vi "HydAcqMaster.vi"() -> ()   [LabVIEW 2022 SP3]
uses:
  ScanningControl/Digitizers/GaGe/-GageUtils/GageGlobals.vi
  <instrlib>/LeCroy Wave Series/LeCroy Wave Series.lvlib
  <vilib>/Utility/file.llb/Read From Spreadsheet File (DBL).vi
panel:
  in  "Erase Data":bool
  out "size(s)":i32[](array[numeric])
  out "Hydrophone Calibration Data":sgl[][](array[numeric]) format="%0.3f"
  out "Calibration Data in use":sgl[](array[numeric])
  in  "Frequency of Interest":u16(ring) items=["1", "2", "3", "4", "5", "6", "7", "8", "9", "10", "11", "12", "13", "14", "15"]
  in  "Hydrophone File":u16(ring) items=["Hydrophone001.txt", "Hydrophone006.txt", "Hydrophone007.txt", "Hydrophone009.txt", "Hydrophone010.txt", "Hydrophone011.txt", "Hydrophone012.txt", "Hydrophone013.txt", "Hydrophone014.txt", "Hydrophone015.txt", "Hydrophone016.txt", "Hydrophone017.txt", "Hydrophone018.txt"]
  in  "LeCroy IP":refnum<visa-resource-name>="VICP::172.25.2.101"
  in  "View Data":bool
  in  "Comment field":string
  in  "Save path":path=path "C:/"
  in  "Scope":bool
  in  "Amp (kV)":sgl
  in  "Init?":bool=TRUE
  out "Handle Cluster 2":T1
  out "Handle Cluster":T1
  in  "FileName":string="test"
  in  "Save Data":bool
  out "Waveforms":sgl[][](graph)
  in  "Sequence":u16=1
  out "Peak Values":cluster{"Z Element Position":sgl[], sgl[]}[](graph)
  in  "Time Out (ms)":dbl=1000.0 min=-1.0
  in  "# Firings":u16=1 min=1
  in  "start scan":bool
  in  "SetDig":bool
  in  "ExitSendCmd":bool
  # "© 2012 Riverside Research Institute"
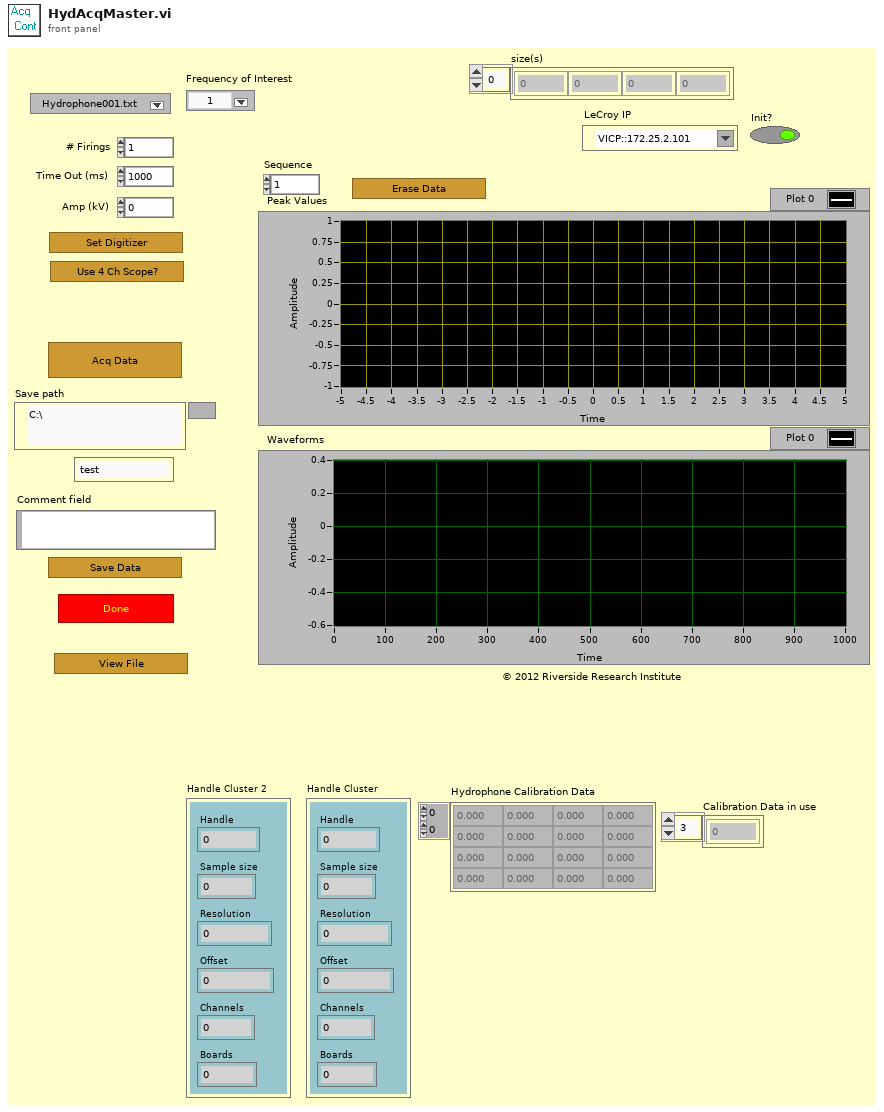
[diagram p1: front panel]
types:
  T1 = cluster{"Handle":u32, "Sample size":u32, "Resolution":i32, "Offset":i32, "Channels":u32, "Boards":u32}
  T2 = enum16{"open", "replace", "create", "open or create", "replace or create", "replace or create with confirmation"}
  T3 = enum16{"big-endian, network order", "native, host order", "little-endian"}
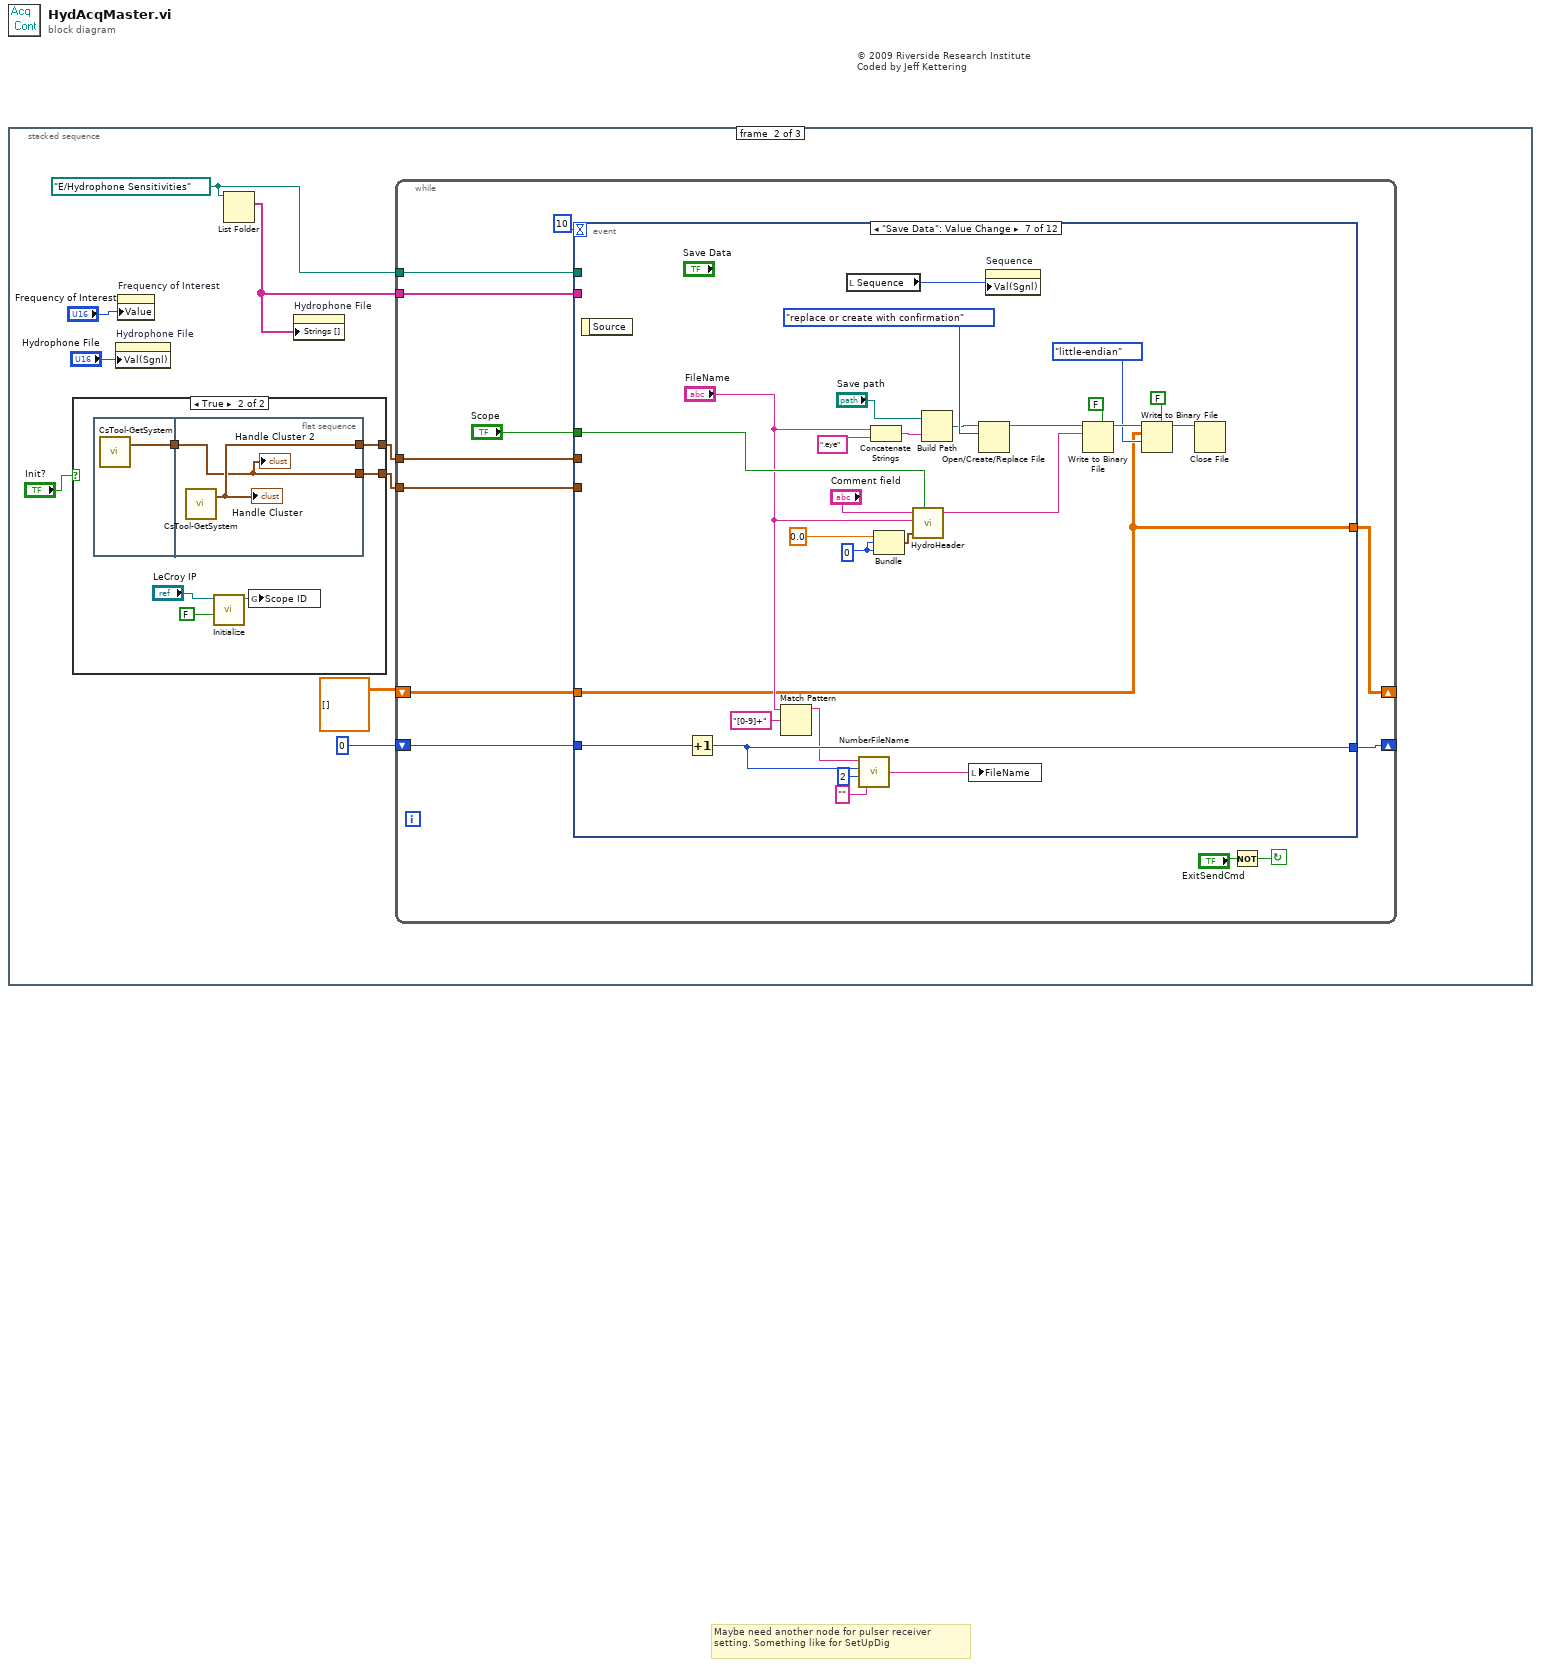
[diagram p0: block diagram]
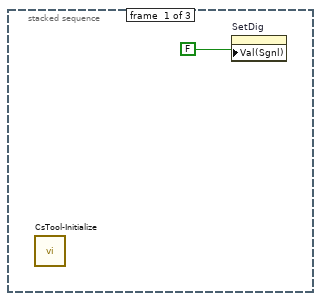
[diagram p2: hidden frame]
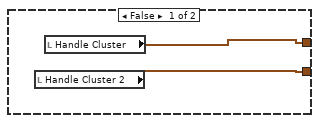
[diagram p3: hidden frame]
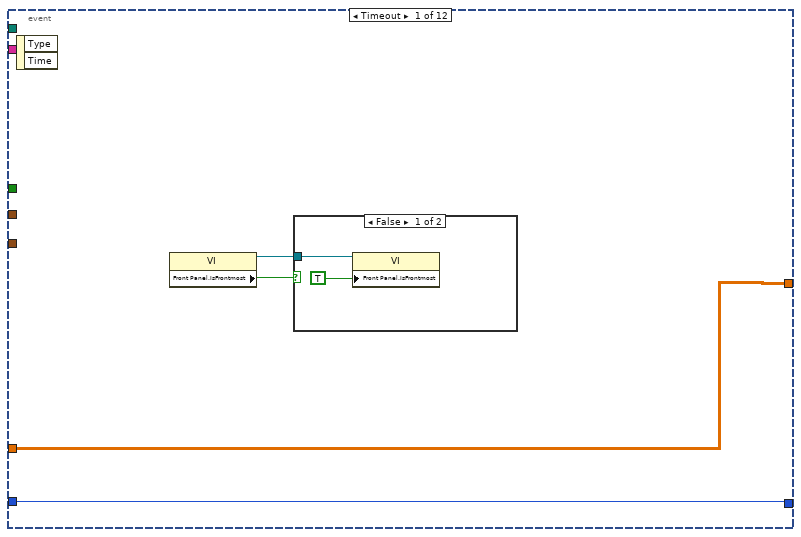
[diagram p4: hidden frame]
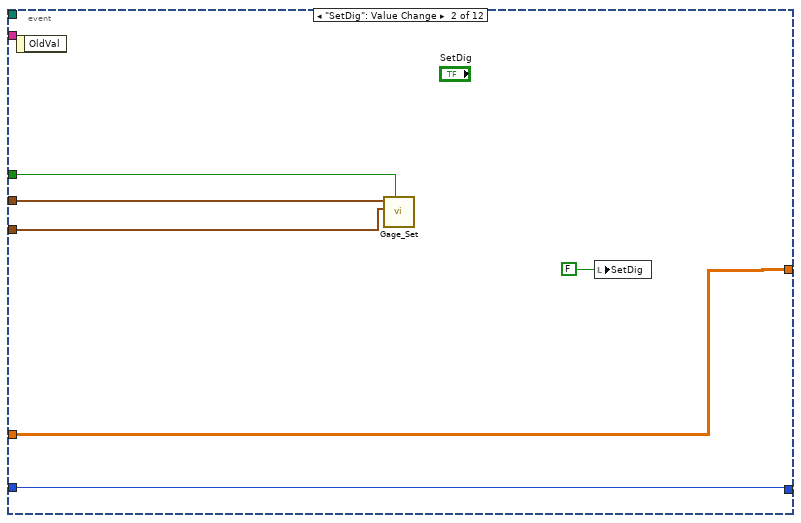
[diagram p6: hidden frame]
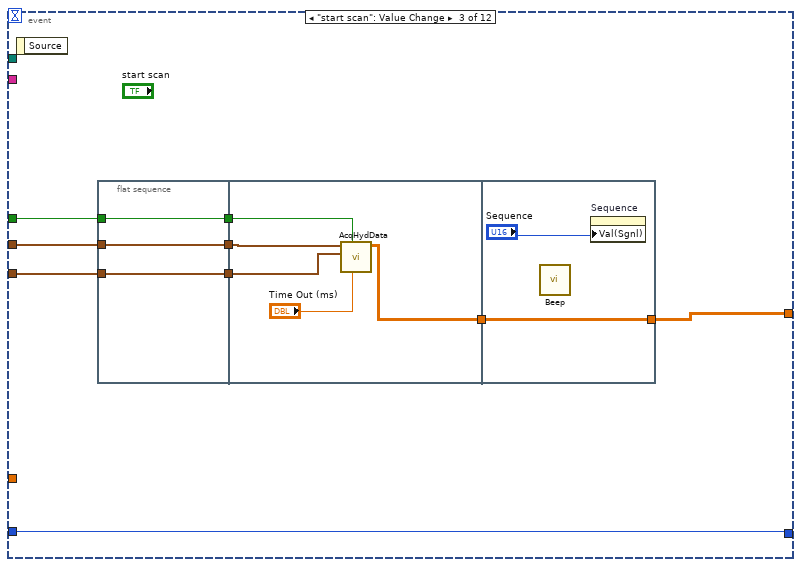
[diagram p7: hidden frame]
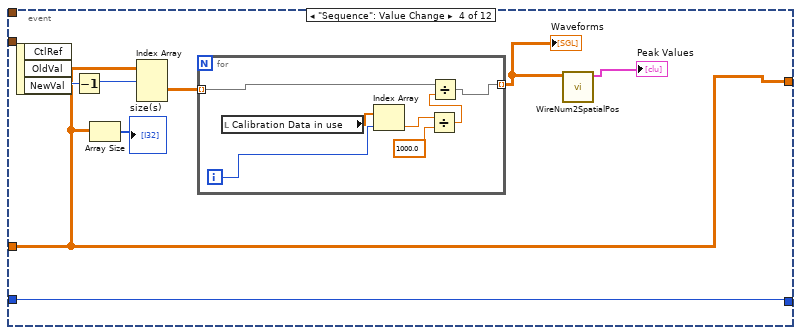
[diagram p8: hidden frame]
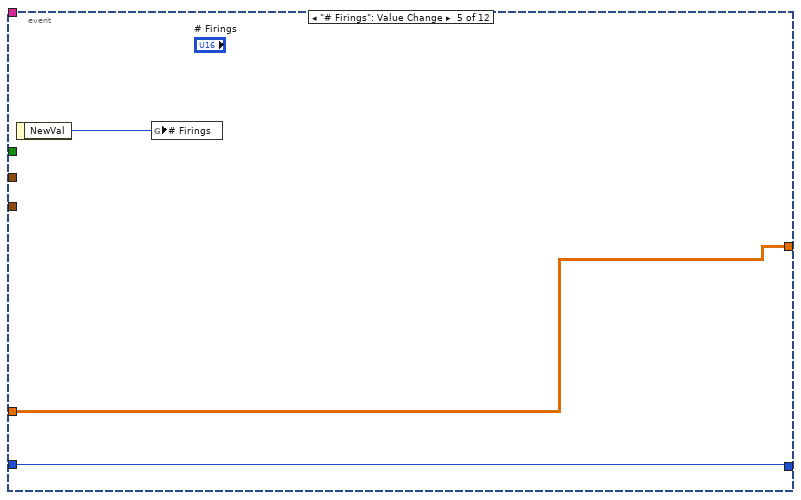
[diagram p9: hidden frame]
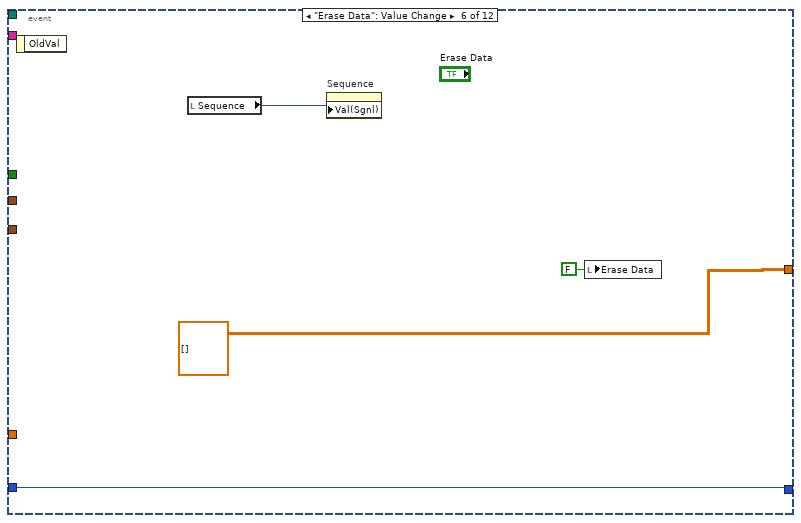
[diagram p10: hidden frame]
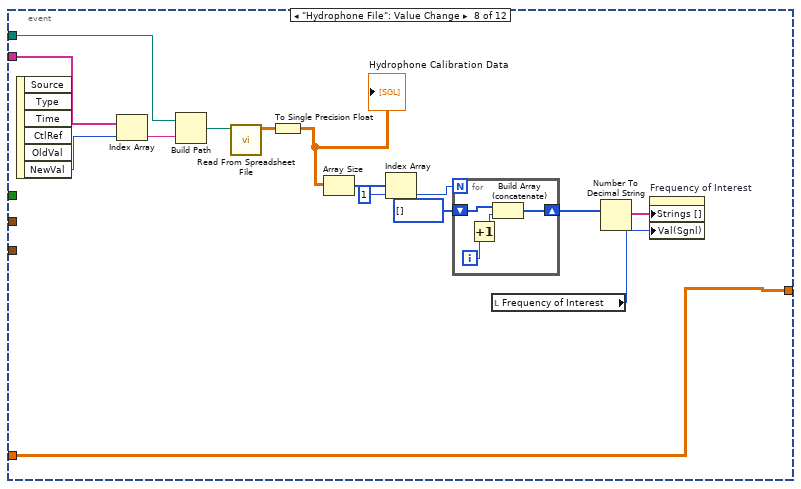
[diagram p11: hidden frame]
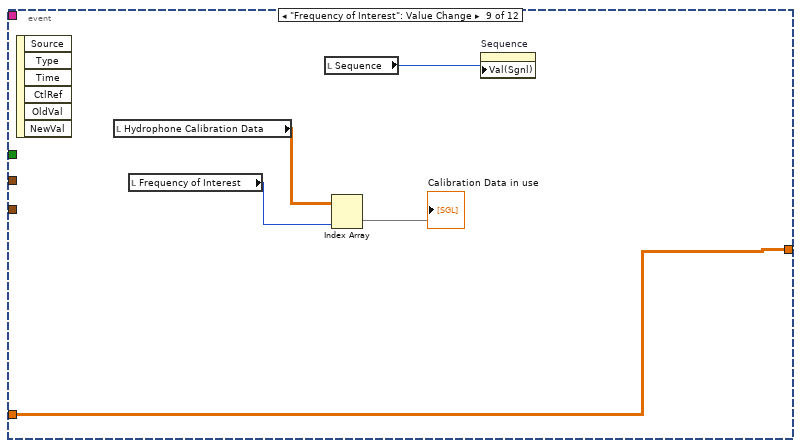
[diagram p12: hidden frame]
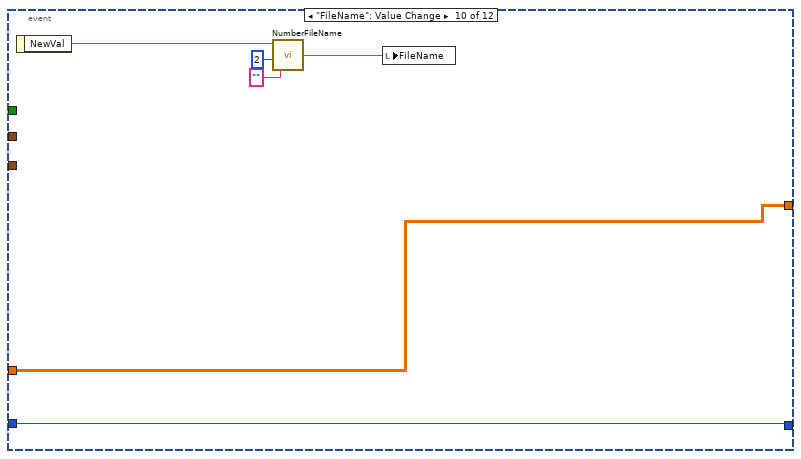
[diagram p13: hidden frame]
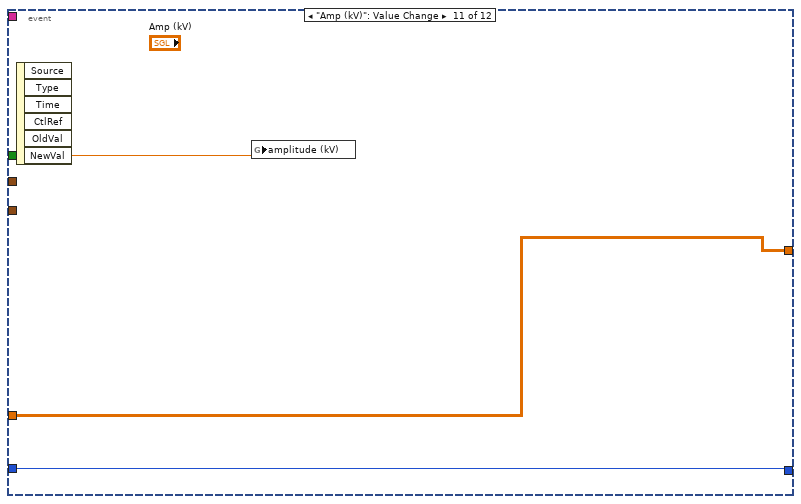
[diagram p14: hidden frame]
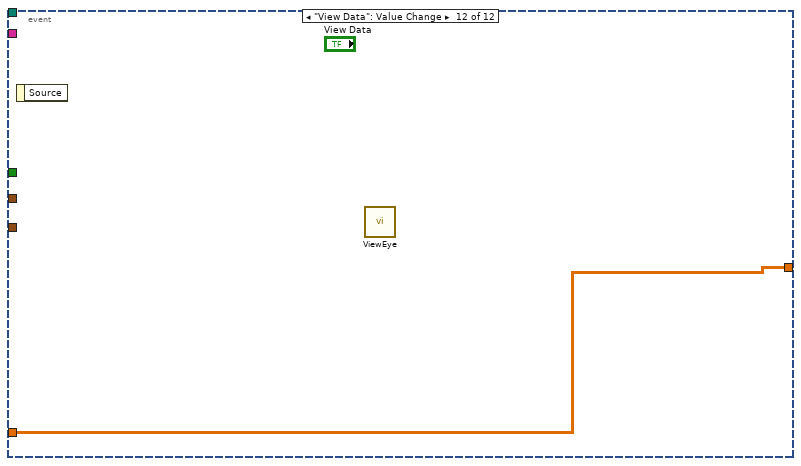
[diagram p15: hidden frame]
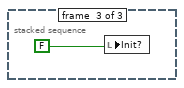
[diagram p16: hidden frame]
diagram:
  # "© 2009 Riverside Research Institute\nCoded by Jeff Kettering"
  # "Maybe need another node for pulser receiver setting. Something like for SetUpDig"
  n1 = stacked-sequence {
    frame #0 {
      n2 = call <userlib>:"CsTool-Initialize.vi"() -> ()  [unwired: 2 out]
      n3 = property on="SetDig" class="Bool (strict)"("Val(Sgnl)"=FALSE) -> ()  [unwired: 2 in, 2 out]
    }
    frame #1 {
      w5 = path "E:/Hydrophone Sensitivities" ("path")
      n4 = case shown="True" "Init?" {
        tunnel: [w12 w17] -> w10
        tunnel: [w11 w16] -> w9
        frame False {
          n5 = local read "Handle Cluster 2"() -> (w11:T1)
          n6 = local read "Handle Cluster"() -> (w12:T1)
        }
        frame True {
          n7 = flat-sequence {
            tunnel: [w19] -> w18
            tunnel: [w21] -> w17
            tunnel: w18 -> [w20]
            tunnel: [w20] -> w16
            frame #0 {
              n8 = call <userlib>:"CsTool-GetSystem.vi"() -> ("Handle Cluster"=w19:T1)  [unwired: 4 in, 1 out]
            }
            frame #1 {
              n9 = call <userlib>:"CsTool-GetSystem.vi"() -> ("Handle Cluster"=w21:T1)  [unwired: 4 in, 1 out]
              "Handle Cluster" <- w21
              "Handle Cluster 2" <- w20
            }
          }
          n10 = call <instrlib>:"Initialize.vi"("Reset? (T: Yes)"=FALSE, "VISA resource name"="LeCroy IP") -> ("VISA resource name out"=w15:refnum<visa-resource-name>)  [unwired: 2 in, 7 out]
          n11 = global write "GageGlobals.vi" "Scope ID"(w15) -> ()
        }
      }
      n12 = property on="Hydrophone File" class="Ring (strict)"("Val(Sgnl)"="Hydrophone File") -> ()  [unwired: 2 in, 2 out]
      n13 = property on="Frequency of Interest" class="Ring (strict)"("Value"="Frequency of Interest") -> ()  [unwired: 2 in, 2 out]
      n14 = List Folder(path=w5) -> (filenames=w2:string[])  [unwired: 3 in, 3 out]
      n15 = property on="Hydrophone File" class="Ring (strict)"("Strings []"=w2) -> ()  [unwired: 2 in, 2 out]
      n16 = while {
        tunnel: w10 -> [w30]
        tunnel: w9 -> [w29]
        shift-right: [w26] -> _
        shift-left: 0 -> [w27]
        tunnel: w2 -> [w25]
        tunnel: w5 -> [w24]
        shift-right: [w23] -> _
        shift-left: sgl[][][] [] ("Data in Volts") -> [w22]
        stop <- w32 continue-if-true
        n17 = event shown="[6] \"Save Data\": Value Change" {
          selector: _ -> [_ _ _ _ _ _ _ _ _ _ _ _]
          dyn-events: _ -> [_ _ _ _ _ _ _ _ _ _ _ _]
          timeout: 10 -> [_ _ _ _ _ _ _ _ _ _ _ _]
          tunnel: w30 -> [_ w45 w54 _ _ _ _ _ _ _ _ _]
          tunnel: w29 -> [_ w44 w53 _ _ _ _ _ _ _ _ _]
          tunnel: "Scope" -> [_ w43 w52 _ _ _ w99 _ _ _ _ _]
          tunnel: w27 -> [w35 w42 w51 w71 w81 w86 w97 _ _ w140 w145 _]
          tunnel: [w35 w42 w51 w71 w81 w86 w94 _ _ w140 w145 _] -> w26
          tunnel: w25 -> [_ _ _ _ _ _ _ w126 _ _ _ _]
          tunnel: w24 -> [_ _ _ _ _ _ _ w124 _ _ _ _]
          tunnel: [w34 w40 w47 w66 w80 sgl[][][] [] ("Data in Volts") w87 w115 w134 w138 w144 w147] -> w23
          tunnel: w22 -> [w34 w40 _ w66 w80 _ w87 w115 w134 w138 w144 w147]
          event Timeout {
            n18 = event-data() -> ()  [unwired: 3 out]
            n19 = property class="VI"() -> (reference out=w37:refnum<vi>, "Front Panel.IsFrontmost"=w36:bool)  [unwired: 2 in, 1 out]
            n20 = case shown="False" w36 {
              tunnel: w37 -> [w39 _]
              frame False {
                n21 = property class="VI"(reference=w39, "Front Panel.IsFrontmost"=TRUE) -> ()  [unwired: 1 in, 2 out]
              }
              frame True {
              }
            }
          }
          event "SetDig": Value Change {
            n22 = event-data() -> ()  [unwired: 2 out]
            n23 = call "Gage_Set.vi"("Scope"=w43, "Handle Cluster 2"=w44, "Handle Cluster 1"=w45) -> ()  [unwired: 9 out]
            n24 = local write "SetDig"(FALSE) -> ()
          }
          event "start scan": Value Change {
            n25 = event-data() -> ()  [unwired: 2 out]
            n26 = flat-sequence {
              tunnel: w52 -> [w55]
              tunnel: w53 -> [w56]
              tunnel: w54 -> [w57]
              tunnel: [w57] -> w50
              tunnel: [w56] -> w49
              tunnel: [w55] -> w48
              tunnel: w50 -> [w62]
              tunnel: w49 -> [w61]
              tunnel: w48 -> [w59]
              tunnel: [w58] -> w46
              tunnel: [w63] -> w47
              tunnel: w46 -> [w63]
              frame #0 {
              }
              frame #1 {
                n27 = call "AcqHydData.vi"("Time Out (ms)"="Time Out (ms)", "Scope"=w59, "Handle Cluster 2"=w61, "Handle Cluster 1"=w62) -> ("Data in Volts"=w58:sgl[][][])  [unwired: 7 out]
              }
              frame #2 {
                n28 = call <vilib>:"Beep.vi"() -> ()  [unwired: 3 in, 9 out]
                n29 = property on="Sequence" class="DigNum (strict)"("Val(Sgnl)"="Sequence") -> ()  [unwired: 2 in, 2 out]
              }
            }
          }
          event "Sequence": Value Change {
            n30 = event-data() -> ("NewVal"=w72:u16)  [unwired: 3 out]
            n31 = Decrement(x=w72) -> (x-1=w65:u16)
            n32 = Array Size(array=w66) -> (size(s)=→"size(s)":i32[])
            n33 = Index Array(array=w66, index (dim 0)=w65) -> (element=w70:sgl[][])  [unwired: 2 in]
            n34 = for {
              tunnel: w70 -> [w78] mode=indexing
              tunnel: [w79] -> w68 mode=indexing
              i -> [w73]
              n35 = local read "Calibration Data in use"() -> (w77:sgl[])
              n36 = Index Array(array=w77, index=w73) -> (element=w75:sgl)
              n37 = Divide(x=w75, y=sgl 1000.0) -> (x/y=w76:sgl)
              n38 = Divide(x=w78, y=w76) -> (x/y=w79:sgl[])
            }
            "Waveforms" <- w68
            n39 = call "WireNum2SpatialPos.vi"("Waveforms"=w68) -> ("Peak Values"=→"Peak Values":cluster{"Z Element Position":sgl[], sgl[]}[])  [unwired: 10 in]
          }
          event "# Firings": Value Change {
            n40 = event-data() -> ("NewVal"=w82:u16)  [unwired: 1 out]
            n41 = global write "GageGlobals.vi" "# Firings"(w82) -> ()
          }
          event "Erase Data": Value Change {
            n42 = event-data() -> ()  [unwired: 2 out]
            n43 = local read "Sequence"() -> (w83:u16)
            n44 = property on="Sequence" class="DigNum (strict)"("Val(Sgnl)"=w83) -> ()  [unwired: 2 in, 2 out]
            n45 = local write "Erase Data"(FALSE) -> ()
          }
          event "Save Data": Value Change {
            w102 = 0
            n46 = event-data() -> ()  [unwired: 2 out]
            n47 = Increment(x=w97) -> (x+1=w94:i32)
            n48 = Match Pattern(string="FileName", regular expression="[0-9]+") -> (before substring=w90:string)  [unwired: 4 out]
            n49 = local read "Sequence"() -> (w89:u16)
            n50 = call "NumberFileName.vi"("String"="", "Digits"=2, "File number"=w94, "file name"=w90) -> ("Numbered File"=w96:string)
            n51 = Concatenate Strings("FileName", ".eye") -> (w105:string)
            n52 = Bundle(0.0, w102, w102) -> (w101:cluster{dbl, i32, i32})  [unwired: 1 out]
            n53 = call "HydroHeader.vi"("Comment"="Comment field", "Scope"=w99, "File Name In"="FileName", "Votage scaling"=w101) -> ("Header String Out"=w113:string)  [unwired: 3 out]
            n54 = Build Path(base path="Save path", name or relative path=w105) -> (appended path=w104:path)
            n55 = local write "FileName"(w96) -> ()
            n56 = Open/Create/Replace File(file path (use dialog)=w104, operation (0:open)=T2."replace or create with confirmation") -> (refnum out=w112:refnum<file>)  [unwired: 1 in, 5 out]
            n57 = property on="Sequence" class="DigNum (strict)"("Val(Sgnl)"=w89) -> ()  [unwired: 2 in, 2 out]
            n58 = Write to Binary File(file (use dialog)=w112, data=w113, 5:FALSE ("prepend array or string size? (T)")) -> (refnum out=w111:refnum<file>)  [unwired: 1 in, 4 out]
            n59 = Write to Binary File(file (use dialog)=w111, data=w87, 5:FALSE ("prepend array or string size? (T)"), 9:T3."little-endian" ("byte order (0:big-endian, network order)")) -> (refnum out=w110:refnum<file>)  [unwired: 1 in, 3 out]
            n60 = Close File(refnum=w110) -> ()  [unwired: 1 in, 2 out]
          }
          event "Hydrophone File": Value Change {
            n61 = event-data() -> ("NewVal"=w125:u16)  [unwired: 6 out]
            n62 = Index Array(array=w126, index=w125) -> (element=w128:string)
            n63 = Build Path(base path=w124, name or relative path=w128) -> (appended path=w127:path)
            n64 = call-poly <vilib>:"Read From Spreadsheet File.vi"("file path (dialog if empty)"=w127) -> ("all rows"=w118:dbl[][])  [unwired: 6 in, 4 out]
            n65 = To Single Precision Float(number=w118) -> (single precision float=w114:sgl[][])
            "Hydrophone Calibration Data" <- w114
            n66 = Array Size(array=w114) -> (size(s)=w123:i32[])
            n67 = Index Array(array=w123, index=1) -> (element=w121:i32)
            n68 = for {
              N: w121 -> [_]
              shift-right: [w131] -> w120
              shift-left: i32[] [] -> [w130]
              i -> [w132]
              n69 = Increment(x=w132) -> (x+1=w129:i32)
              n70 = Build Array (concatenate)(w130, w129) -> (w131:i32[])
            }
            n71 = local read "Frequency of Interest"() -> (w116:u16)
            n72 = Number To Decimal String(number=w120) -> (decimal integer string=w119:string[])  [unwired: 1 in]
            n73 = property on="Frequency of Interest" class="Ring (strict)"("Strings []"=w119, "Val(Sgnl)"=w116) -> ()  [unwired: 2 in, 2 out]
          }
          event "Frequency of Interest": Value Change {
            n74 = event-data() -> ()  [unwired: 7 out]
            n75 = local read "Hydrophone Calibration Data"() -> (w135:sgl[][])
            n76 = local read "Frequency of Interest"() -> (w136:u16)
            n77 = local read "Sequence"() -> (w133:u16)
            n78 = Index Array(array=w135, index (col)=w136) -> (element=→"Calibration Data in use":sgl[])  [unwired: 1 in]
            n79 = property on="Sequence" class="DigNum (strict)"("Val(Sgnl)"=w133) -> ()  [unwired: 2 in, 2 out]
          }
          event "FileName": Value Change {
            n80 = event-data() -> ("NewVal"=w142:string)  [unwired: 1 out]
            n81 = call "NumberFileName.vi"("String"="", "Digits"=2, "file name"=w142) -> ("Numbered File"=w141:string)  [unwired: 1 in]
            n82 = local write "FileName"(w141) -> ()
          }
          event "Amp (kV)": Value Change {
            n83 = event-data() -> ("NewVal"=w146:sgl)  [unwired: 6 out]
            n84 = global write "GageGlobals.vi" "amplitude (kV)"(w146) -> ()
          }
          event "View Data": Value Change {
            n85 = event-data() -> ()  [unwired: 2 out]
            n86 = call "ViewEye.vi"() -> ()  [unwired: 1 out]
          }
        }
        n87 = Not(x="ExitSendCmd") -> (.not. x?=w32:bool)
      }
    }
    frame #2 {
      n88 = local write "Init?"(FALSE) -> ()
    }
  }
